vi "Untitled 1.vi"() -> ()   [LabVIEW 2015]
uses:
  <vilib>/Analysis/baseanly.llb/Mean (DBL).vi
  <vilib>/measure/madcrms.llb/Basic Averaged DC-RMS for N Chan.vi
  <vilib>/Analysis/NI_AALBase.lvlib
  <vilib>/measure/NI_MAPro.lvlib
panel:
  out "RMS values":dbl[](array[numeric]) format="%.2p"
  in  "stop":bool
  out "mean":dbl format="%0.2f"
  out "data":dynamicdata(graph)
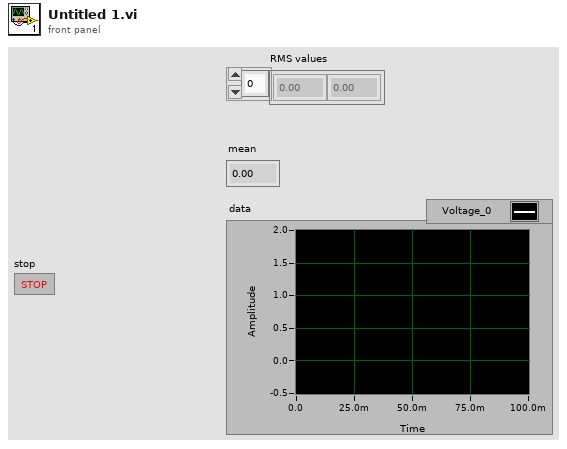
[diagram p1: front panel]
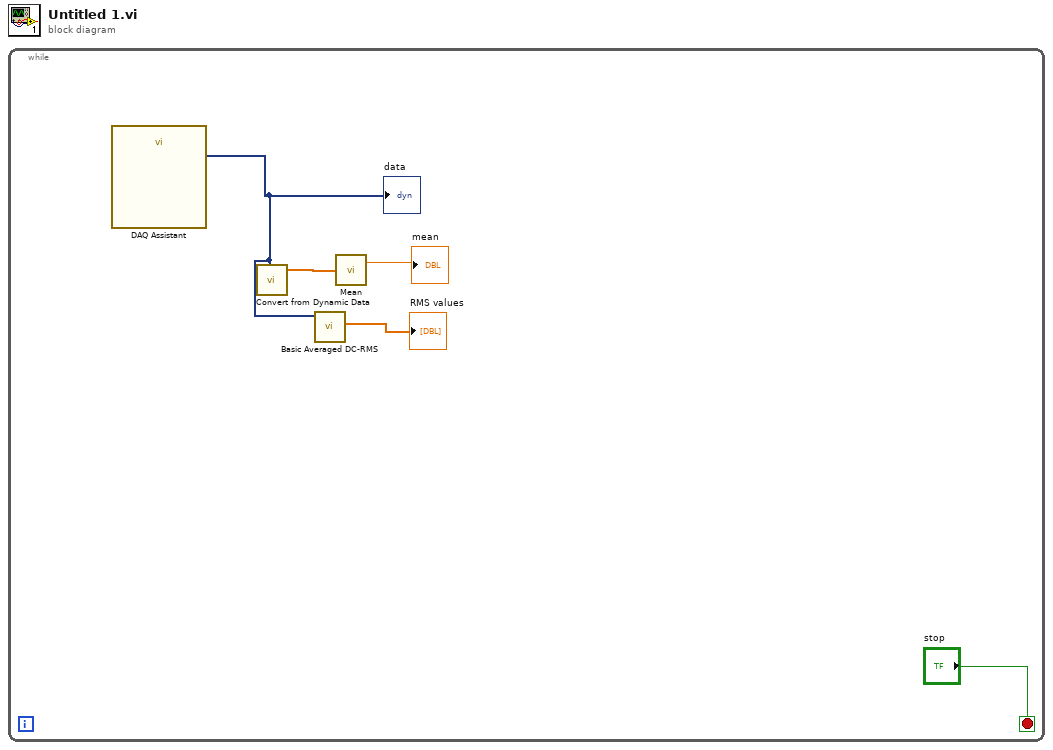
[diagram p0: block diagram]
diagram:
  n1 = while {
    stop <- "stop" stop-if-true
    n2 = call "DAQ Assistant"() -> ("data"=w2:dynamicdata)  [unwired: 17 in, 2 out]
    "data" <- w2
    n3 = call "Convert from Dynamic Data"("Dynamic Data Type"=w2) -> ("Array"=w5:dbl[])  [unwired: 3 in]
    n4 = call-poly <vilib>:"Basic Averaged DC-RMS.vi"("signals in"=w2) -> ("RMS values"=→"RMS values":dbl[])  [unwired: 7 in, 3 out]
    n5 = call-poly <vilib>:"Mean.vi"("X"=w5) -> ("mean"=→"mean":dbl)  [unwired: 1 out]
  }
